vi "Write Stimulus Parameter.vi"(8 "error in (no error)":errorcluster, 10 "Stimulus Parameters":T1, 11 "Data Analyser Report in":refnum<class "Data Analyser Report.lvclass">) -> (0 "error out":errorcluster, 3 "Data Analyser Report out":refnum<class "Data Analyser Report.lvclass">)   [LabVIEW 2016, in "Data Analyser Report.lvclass"]
uses:
  Data Analyser Report.lvclass
  C:/Users/w.figtree/Desktop/Work/4. Projects/3. In Progress Engineering Projects/EMA/src/core/Classes/Excel Interface/Excel Sheet/Excel Sheet.lvclass
  Excel Interface/Excel Sheet/Write to Cell - Int.vi
  Excel Interface/Excel Sheet/Write to Cell - Dbl.vi
  Excel Interface/Excel Sheet/Excel Sheet.lvclass
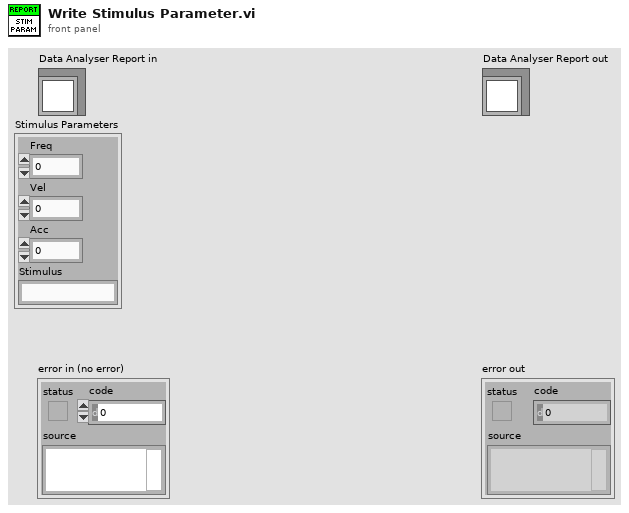
[diagram p1: front panel]
types:
  T1 = cluster{"Freq":dbl, "Vel":i32, "Acc":i32, "Stimulus":string}
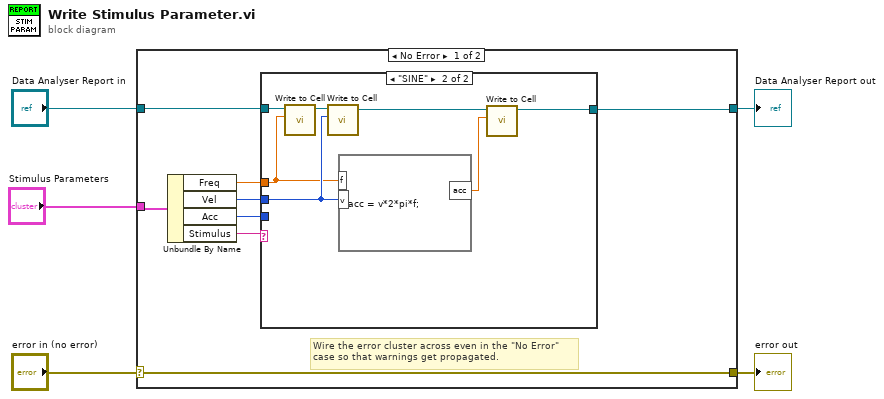
[diagram p0: block diagram]
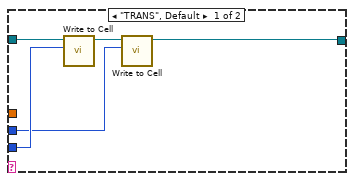
[diagram p2: hidden frame]
diagram:
  n1 = case shown="No Error" "error in (no error)" {
    selector: "error in (no error)" -> [w13 w27]
    tunnel: [w13 w27] -> w4
    tunnel: [w6 w26] -> w2
    tunnel: "Data Analyser Report in" -> [w10 w26]
    tunnel: "Stimulus Parameters" -> [w12 _]
    frame No Error {
      # "Wire the error cluster across even in the \"No Error\"\ncase so that warnings get propagated."
      n2 = Unbundle By Name(w12) -> ("Freq"=w9:dbl, "Vel"=w8:i32, "Acc"=w7:i32, "Stimulus"=w11:string)
      n3 = case shown="\"SINE\"" w11 {
        tunnel: w10 -> [w18 w25]
        tunnel: w9 -> [_ w22]
        tunnel: w8 -> [w15 w23]
        tunnel: w7 -> [w17 _]
        tunnel: [w14 w19] -> w6
        frame "TRANS", Default {
          n4 = call-poly "Write to Cell.vi"("Value"=w17, "Excel Sheet in"=w18) -> ("Excel Sheet out"=w16:refnum<class "Data Analyser Report.lvclass">)  [unwired: 9 in]
          n5 = call-poly "Write to Cell.vi"("Value"=w15, "Excel Sheet in"=w16) -> ("Excel Sheet out"=w14:refnum<class "Data Analyser Report.lvclass">)  [unwired: 9 in]
        }
        frame "SINE" {
          n6 = call-poly "Write to Cell.vi"("Value"=w22, "Excel Sheet in"=w25) -> ("Excel Sheet out"=w24:refnum<class "Data Analyser Report.lvclass">)  [unwired: 9 in]
          n7 = call-poly "Write to Cell.vi"("Value"=w23, "Excel Sheet in"=w24) -> ("Excel Sheet out"=w20:refnum<class "Data Analyser Report.lvclass">)  [unwired: 9 in]
          n8 = formula code="acc = v*2*pi*f;"("v"=w23, "f"=w22) -> ("acc"=w21:dbl)
          n9 = call-poly "Write to Cell.vi"("Value"=w21, "Excel Sheet in"=w20) -> ("Excel Sheet out"=w19:refnum<class "Data Analyser Report.lvclass">)  [unwired: 9 in]
        }
      }
    }
    frame Error {
    }
  }
  "error out" <- w4
  "Data Analyser Report out" <- w2
